vi "求排列.vi"(1 "k":u32=100, 2 "n":u32=100) -> (0 "nPk":dbl)   [LabVIEW 2012]
doc: "功能：\n\n利用化简组合公式求组合。\n\n公式：\n\nC(n,k)=n!/(k!*(n-k)!\n\n根据阶乘的定义，n!可以被k!或者（n-k）的阶乘约分，因此可以选择k和n-k中较大的进行约分，极大地减少了循环次数，避免了阶乘溢出的问题。\n\n\nCSXCS_366创建"
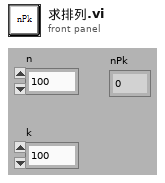
[diagram p1: front panel]
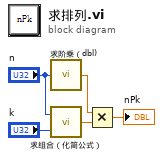
[diagram p0: block diagram]
diagram:
  n1 = call "求阶乘（dbl).vi"("Num"="n") -> ("Fract"=w3:dbl)
  n2 = call "求组合（化简公式）.vi"("k"="k", "n"="n") -> ("C(n,k)"=w2:dbl)
  n3 = Multiply(x=w3, y=w2) -> (x*y=→"nPk":dbl)
